vi "RW utf-8.vi"() -> ()   [LabVIEW 2020]
panel:
  out "utf-8 Encoded":string
  out "Decoded":string
  out "Original":string
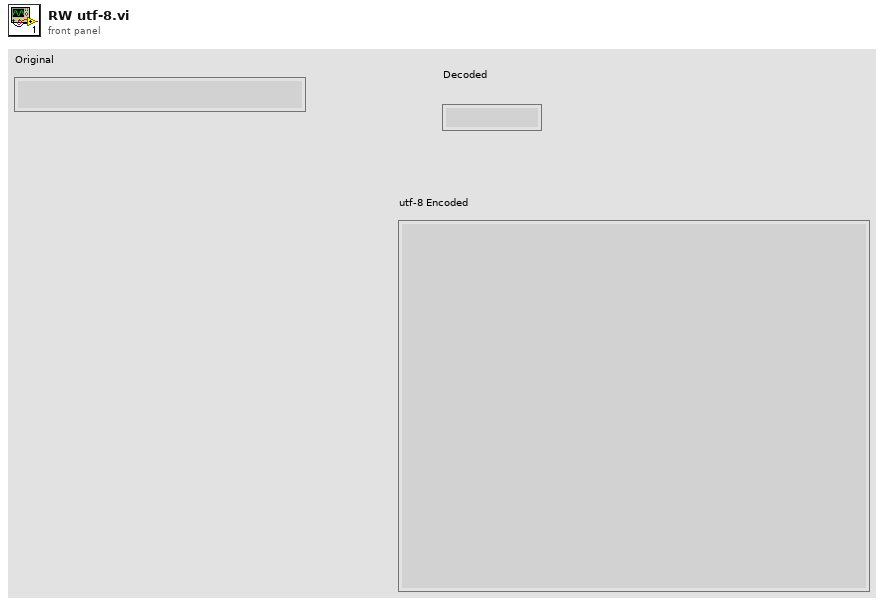
[diagram p1: front panel]
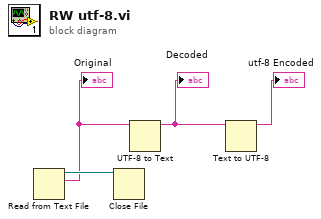
[diagram p0: block diagram]
diagram:
  n1 = Read from Text File() -> (refnum out=w4:refnum<file>, text=w3:string)  [unwired: 4 in, 2 out]
  "Original" <- w3
  n2 = Close File(refnum=w4) -> ()  [unwired: 1 in, 2 out]
  n3 = UTF-8 to Text(11:w3) -> (3:w2:string)  [unwired: 2 in, 1 out]
  "Decoded" <- w2
  n4 = Text to UTF-8(11:w2) -> (3:→"utf-8 Encoded":string)  [unwired: 2 in, 1 out]
